vi "二维数组查找元素_布尔.vi"(6 "元素":bool=TRUE, 8 "error in (no error)":errorcluster caption="错误输入（无错误）", 11 "数组":bool[][](array[boolean])) -> (0 "error out":errorcluster caption="错误输出", 3 "索引数组":i32[][](array[numeric]))   [LabVIEW 2014]
doc: "该模板用于创建子VI。"
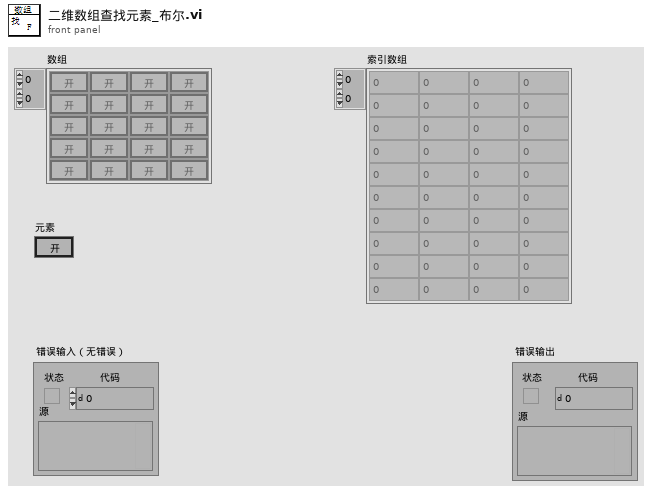
[diagram p1: front panel]
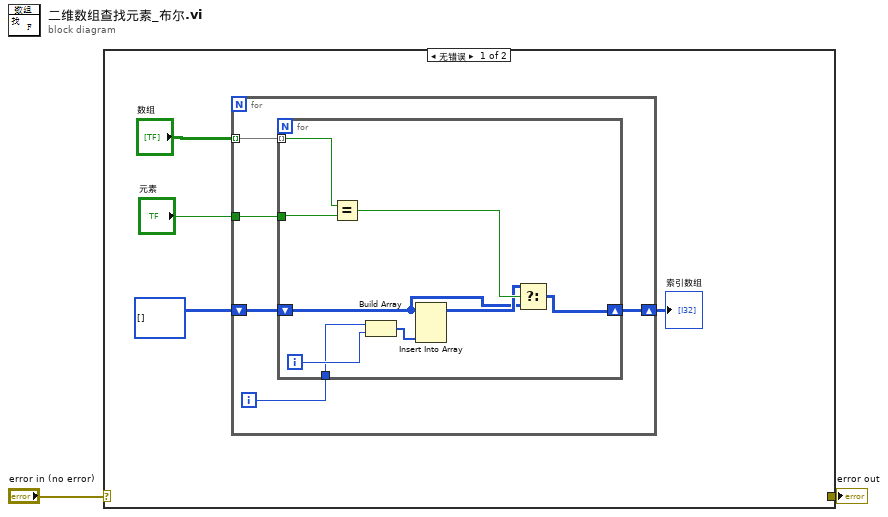
[diagram p0: block diagram]
diagram:
  n1 = case shown="无错误" "error in (no error)" {
    selector: "error in (no error)" -> [_ w21]
    tunnel: [_ w21] -> w1
    frame No Error {
      n2 = for {
        tunnel: "数组" -> [w11] mode=indexing
        tunnel: "元素" -> [w10]
        shift-right: [w7] -> w3
        shift-left: i32[][] [] -> [w8]
        i -> [w9]
        n3 = for {
          tunnel: w11 -> [w20] mode=indexing
          tunnel: w10 -> [w19]
          tunnel: w9 -> [w13]
          shift-right: [w15] -> w7
          shift-left: w8 -> [w16]
          i -> [w14]
          n4 = Equal?(x=w20, y=w19) -> (x = y?=w18:bool)
          n5 = Build Array(w13, w14) -> (w12:i32[])
          n6 = Insert Into Array(array=w16, new element=w12) -> (w17:i32[][])  [unwired: 2 in]
          n7 = Select(t=w17, s=w18, f=w16) -> (s? t:f=w15:i32[][])
        }
      }
      "索引数组" <- w3
    }
    frame Error {
    }
  }
  "error out" <- w1
